vi "Connect(config).vi"(8 "error in (no error)":errorcluster, 11 "path to client config":path) -> (0 "error out":errorcluster, 3 "Client out":refnum<class "Client.lvclass">)   [LabVIEW 2017, in "opcua.lvlib" / "Client.lvclass"]
uses:
  Client.lvclass
  Client.lvclass/Client.ctl
  opcua32.dll
  opcua.lvlib
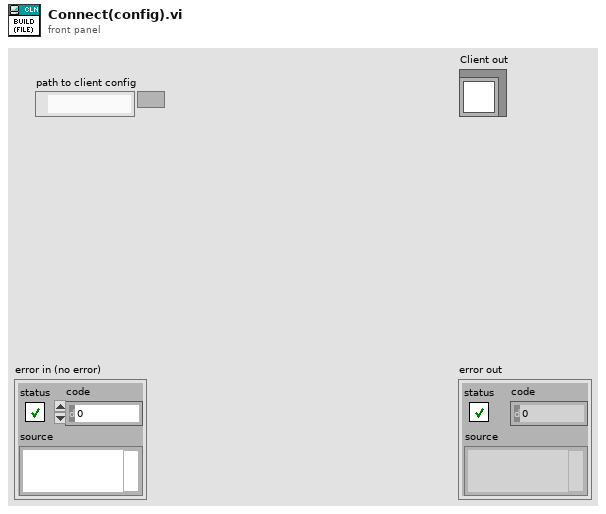
[diagram p1: front panel]
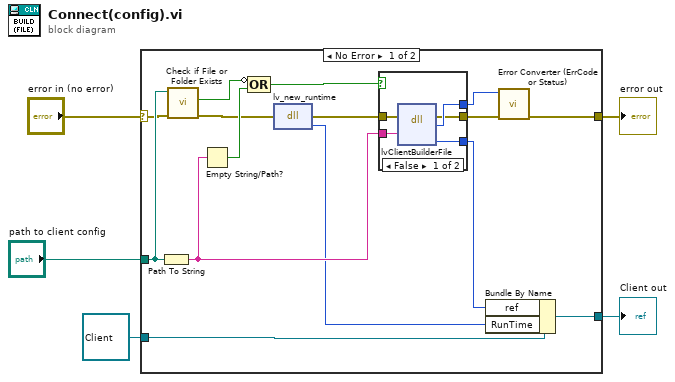
[diagram p0: block diagram]
diagram:
  n1 = case shown="No Error" "error in (no error)" {
    selector: "error in (no error)" -> [w8 w27]
    tunnel: [w16 w27] -> w4
    tunnel: [w17 w28] -> w2
    tunnel: refnum<class "Client.lvclass"> refnum ("Client in") -> [w18 w28]
    tunnel: "path to client config" -> [w13 _]
    frame No Error {
      n2 = Path To String(path=w13) -> (string=w11:string)
      n3 = call <vilib>:"Check if File or Folder Exists.vi"("error in (no error)"=w8, "path"=w13) -> ("error out"=w7:errorcluster, "file or folder exists?"=w14:bool)  [unwired: 7 in, 1 out]
      n4 = Empty String/Path?(string/path=w11) -> (empty?=w15:bool)
      n5 = Compound Arithmetic op=OR(invert w14, w15) -> (w12:bool)
      n6 = dll-call lib="C:/Users/108003658/OneDrive - Baker Hughes/Desktop/opcua-0_2_0/opcua-lvlib/opcua*.dll" fn="lv_new_runtime"(error in=w7) -> (error out=w10:errorcluster, "return type"=w9:u64)  [unwired: 2 in, 1 out]
      n7 = case shown="False" w12 {
        tunnel: [w25 _] -> w20
        tunnel: w10 -> [w24 w26]
        tunnel: [w23 _] -> w19
        tunnel: w11 -> [w22 _]
        tunnel: [w21 w26] -> w6
        frame False {
          n8 = dll-call lib="C:/Users/108003658/OneDrive - Baker Hughes/Desktop/opcua-0_2_0/opcua-lvlib/opcua*.dll" fn="lvClientBuilderFile"(error in=w24, "config_file"=w22) -> (error out=w21:errorcluster, "return type"=w23:i32, "client_ref"=w25:u64)  [unwired: 4 in, 1 out]
        }
        frame True {
        }
      }
      n9 = Bundle By Name(cluster=w18, "ref"=w20, "RunTime"=w9) -> (w17:refnum<class "Client.lvclass">)
      n10 = call "Error Converter (ErrCode or Status).vi"("error in (no error)"=w6, "error code"=w19) -> ("error out"=w16:errorcluster)  [unwired: 9 in]
    }
    frame Error {
    }
  }
  "error out" <- w4
  "Client out" <- w2
